vi "Update BrowerComponent.vi"(8 "error in (no error)":errorcluster, 9 "AbstractBuilder":refnum<class "AbstractBuilder.lvclass">, 10 "BrowerComponentID(\"\")":string, 11 "BrowerController in":refnum<class "BrowerController.lvclass">) -> (0 "error out":errorcluster, 3 "BrowerController out":refnum<class "BrowerController.lvclass">)   [LabVIEW 2015, in "BrowerController.lvclass"]
uses:
  BrowerController.lvclass
  Models/BrowerBuilder/AbstractBuilder/AbstractBuilder.lvclass
  BrowerController.lvclass/BrowerController.ctl
  Models/BrowerTree/Type Definition/Symbol Index.ctl
  Models/BrowerComponent/BrowerComponent/BrowerComponent.lvclass
  Models/BrowerTree/BrowerTree.lvclass
  Models/BrowerBuilder/BrowerGuidencer/BrowerGuidencer.lvclass
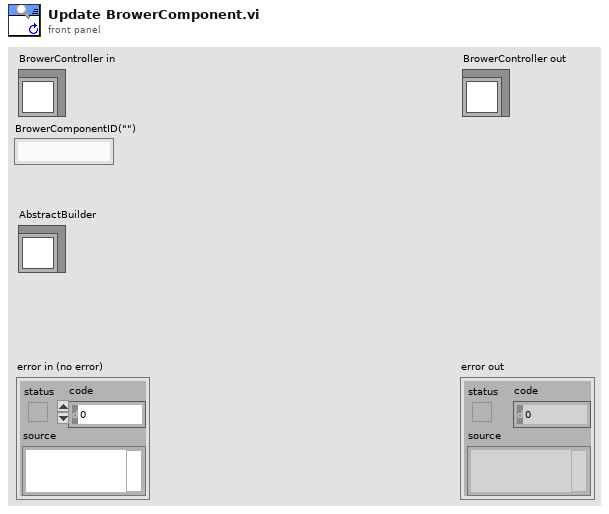
[diagram p1: front panel]
types:
  T1 = typedef "BrowerTree.lvclass/Symbol Index.ctl" = enum16{"PC", "Project", "Module", "DebugTask", "Communication"}
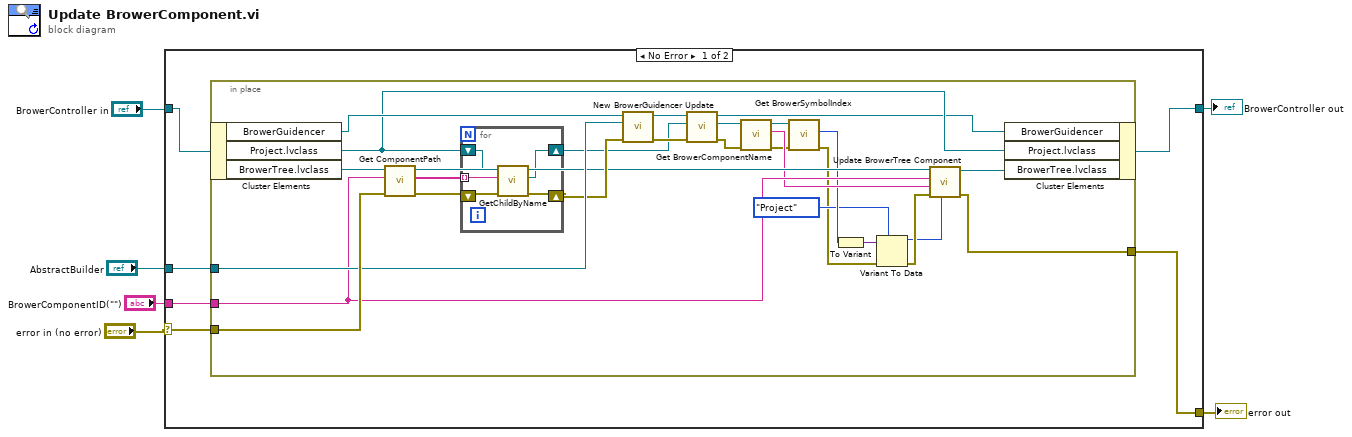
[diagram p0: block diagram]
diagram:
  n1 = case shown="No Error" "error in (no error)" {
    selector: "error in (no error)" -> [w12 w46]
    tunnel: [w7 w46] -> w4
    tunnel: [w9 w45] -> w1
    tunnel: "BrowerController in" -> [w10 w45]
    tunnel: "BrowerComponentID(\"\")" -> [w11 _]
    tunnel: "AbstractBuilder" -> [w8 _]
    frame No Error {
      n2 = in-place {
        in-place-border: w12 -> [w38]
        in-place-border: w11 -> [w28]
        in-place-border: w8 -> [w34]
        in-place-border: [w21] -> w7
        n3 = in-place-cluster #1(w10) -> ("BrowerGuidencer"=w35:refnum<class "BrowerGuidencer.lvclass">, "Project.lvclass"=w20:refnum<class "BrowerComponent.lvclass">, "BrowerTree.lvclass"=w39:refnum<class "BrowerTree.lvclass">)
        n4 = call "Get ComponentPath.vi"("error in (no error)"=w38, "BrowerComponentID(\"\")"=w28, "BrowerTree in"=w39) -> ("error out"=w36:errorcluster, "Navigate Tree:Get Paths"=w37:string[], "BrowerTree out"=w29:refnum<class "BrowerTree.lvclass">)  [unwired: 6 in]
        n5 = for {
          tunnel: w37 -> [w43] mode=indexing
          shift-right: [w41] -> w30
          shift-left: w20 -> [w42]
          shift-right: [w40] -> w33
          shift-left: w36 -> [w44]
          n6 = call-dynamic "GetChildByName.vi"("error in (no error)"=w44, "BrowerComponentID(\"\")"=w43, "reference in"=w42) -> ("error out"=w40:errorcluster, "BrowerComponent"=w41:refnum<class "BrowerComponent.lvclass">)  [unwired: 6 in, 1 out]
        }
        n7 = call "New BrowerGuidencer.vi"("error in (no error)"=w33, "AbstractBuilder"=w34, "reference in"=w35) -> ("error out"=w31:errorcluster, "reference out"=w32:refnum<class "BrowerGuidencer.lvclass">)  [unwired: 7 in]
        n8 = call "Update.vi"("error in (no error)"=w31, "BrowerComponent"=w30, "BrowerGuidencer in"=w32) -> ("error out"=w26:errorcluster, "BrowerComponent out"=w27:refnum<class "BrowerComponent.lvclass">, "BrowerGuidencer out"=w19:refnum<class "BrowerGuidencer.lvclass">)  [unwired: 6 in]
        n9 = call "Get BrowerComponentName.vi"("error in (no error)"=w26, "BrowerComponent in"=w27) -> ("error out"=w23:errorcluster, "ComponentName"=w25:string, "BrowerComponent out"=w24:refnum<class "BrowerComponent.lvclass">)  [unwired: 7 in]
        n10 = call "Get BrowerSymbolIndex.vi"("error in (no error)"=w23, "BrowerComponent in"=w24) -> ("error out"=w15:errorcluster, "SymbolIndex"=w18:i32)  [unwired: 7 in, 1 out]
        n11 = To Variant(anything=w18) -> (Variant=w17:variant)
        n12 = Variant To Data(error in=w15, type=Symbol_Index."Project" ("SymbolIndex"), Variant=w17) -> (data=w13:T1, error out=w14:errorcluster)
        n13 = call "Update BrowerTree Component.vi"("SymbolIndex"=w13, "error in (no error)"=w14, "BrowerComponentNewName(\"\")"=w25, "BrowerComponentID(\"\")"=w28, "BrowerTree in"=w29) -> ("error out"=w21:errorcluster, "BrowerTree out"=w22:refnum<class "BrowerTree.lvclass">)  [unwired: 5 in]
        n14 = in-place-cluster #1("BrowerGuidencer"=w19, "Project.lvclass"=w20, "BrowerTree.lvclass"=w22) -> (w9:refnum<class "BrowerController.lvclass">)
      }
    }
    frame Error {
    }
  }
  "error out" <- w4
  "BrowerController out" <- w1
